vi "monitor.vi"(0 "HIFU_TCP in":refnum<k5>, 1 "HIFU":bool, 2 "chn num":i16=64, 3 "error in (no error)":errorcluster, 4 "sequence":u32) -> (5 "SEQ out":u32, 6 "current":dbl[](array[numeric]), 7 "HIFU_TCP out":refnum<k5>, 8 "voltage":dbl[](array[numeric]), 9 "OK?":bool, 10 "error out":errorcluster)   [LabVIEW 2016]
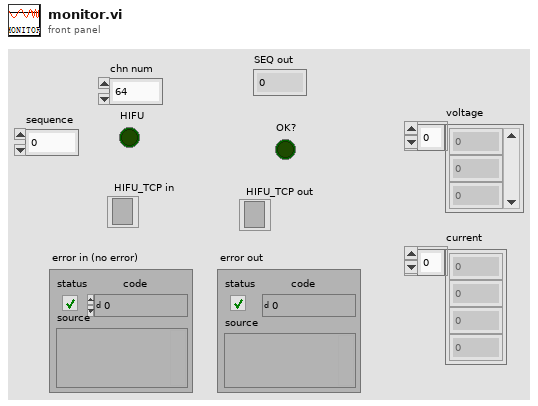
[diagram p1: front panel]
types:
  T1 = enum8{"SET_FREQ", "SET_VOLT", "SET_CHANNEL_VOLT", "SET_PHASE", "START_HEAT", "STOP_HEAT", "CHANNEL_CTRL_SINGLE", "CHANNEL_CTRL_ALL", "READ_VOLT_SET", "READ_VOLT_SET_RSP", "READ_CURRENT_VOLT", "READ_CURRENT_VOLT_RSP", "READ_PHASE", "READ_PHASE_RSP", "READ_HEATTIME_LEFT", "READ_HEATTIME_LEFT_RSP", "EXEC_RSP"}
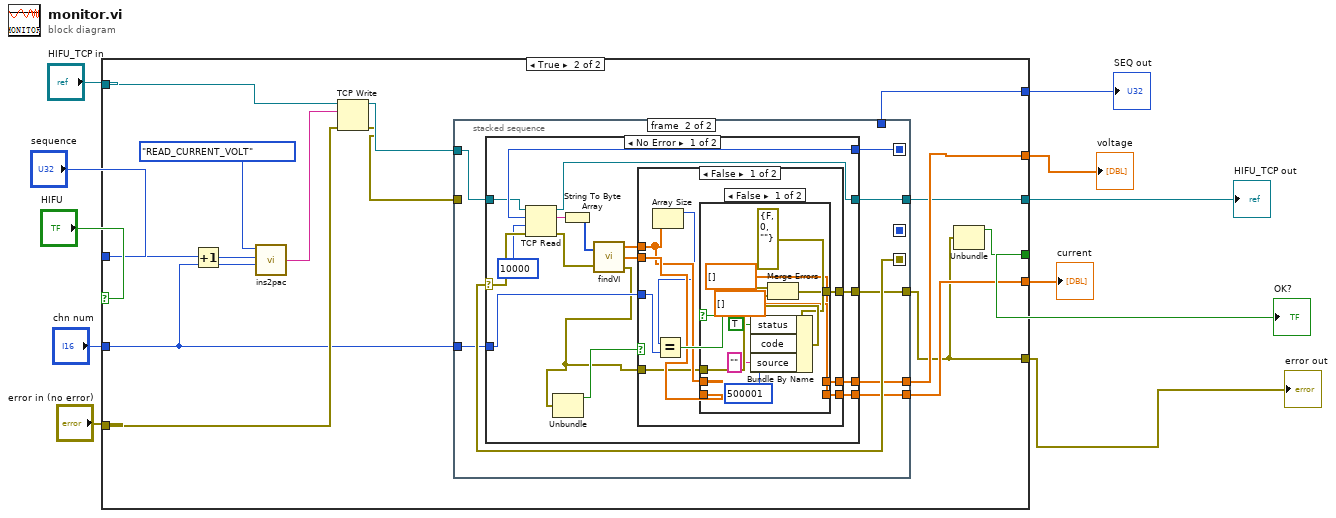
[diagram p0: block diagram]
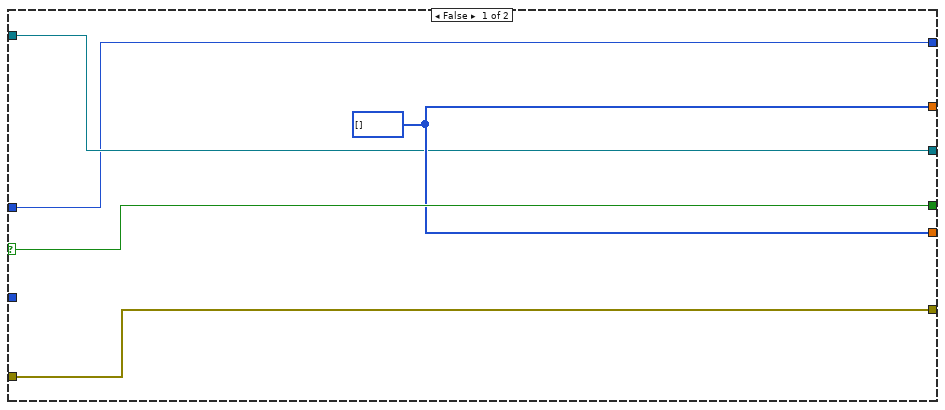
[diagram p2: hidden frame]
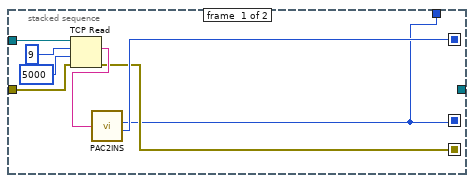
[diagram p3: hidden frame]
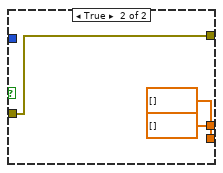
[diagram p5: hidden frame]
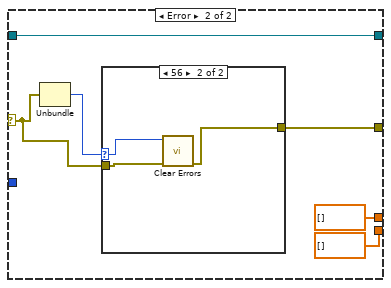
[diagram p6: hidden frame]
diagram:
  n1 = case shown="True" "HIFU" {
    selector: "HIFU" -> [w16 _]
    tunnel: "error in (no error)" -> [w15 w29]
    tunnel: [w14 w24] -> w9
    tunnel: [w14 w25] -> w8
    tunnel: [w15 w22] -> w1
    tunnel: [w16 w21] -> w7
    tunnel: "chn num" -> [_ w26]
    tunnel: "HIFU_TCP in" -> [w13 w31]
    tunnel: "sequence" -> [w12 w20]
    tunnel: [w13 w23] -> w3
    tunnel: [w12 w18] -> w2
    frame False {
      w14 = i32[] []
    }
    frame True {
      n2 = Increment(x=w20) -> (x+1=w19:u32)
      n3 = call "ins2pac.vi"("chn num"=w26, "SEQUENCE"=w19, "TYPE"=T1."READ_CURRENT_VOLT") -> ("PACKET"=w30:string)  [unwired: 1 in]
      n4 = TCP Write(connection ID=w31, data in=w30, error in (no error)=w29) -> (connection ID out=w28:refnum<k5>, error out=w27:errorcluster)  [unwired: 1 in, 1 out]
      n5 = stacked-sequence {
        seq-local: [w34 _] -> [_ w40]
        seq-local: [w32 _] -> [_ _]
        seq-local: [w33 _] -> [_ w46]
        tunnel: w28 -> [w39 w47]
        tunnel: w27 -> [w36 _]
        tunnel: w26 -> [_ w45]
        tunnel: [_ w44] -> w25
        tunnel: [_ w43] -> w24
        tunnel: [_ w42] -> w22
        tunnel: [_ w41] -> w23
        tunnel: [w32 _] -> w18
        frame #0 {
          n6 = TCP Read(connection ID=w39, bytes to read=9, error in (no error)=w36, 9:5000 ("timeout ms (25000)")) -> (data out=w35:string, error out=w33:errorcluster)  [unwired: 1 in, 1 out]
          n7 = call "PAC2INS.vi"("PACKET"=w35) -> ("SEQUENCE"=w32:u32, "LENGTH"=w34:u32)  [unwired: 2 out]
        }
        frame #1 {
          n8 = case shown="No Error" w46 {
            selector: w46 -> [w61 w89]
            tunnel: w40 -> [w63 _]
            tunnel: w47 -> [w62 w90]
            tunnel: w45 -> [w54 _]
            tunnel: [w53 dbl[] [] ("V")] -> w44
            tunnel: [w52 dbl[] [] ("I")] -> w43
            tunnel: [w51 w91] -> w42
            tunnel: [w50 w90] -> w41
            frame No Error {
              n9 = TCP Read(connection ID=w62, bytes to read=w63, error in (no error)=w61, 9:10000 ("timeout ms (25000)")) -> (connection ID out=w50:refnum<k5>, data out=w59:string, error out=w57:errorcluster)  [unwired: 1 in]
              n10 = String To Byte Array(string=w59) -> (unsigned byte array=w58:u8[])
              n11 = call "findVI.vi"("Array"=w58, "error in (no error)"=w57) -> ("V"=w56:dbl[], "I"=w55:dbl[], "error out"=w48:errorcluster)
              n12 = Unbundle(w48) -> ("status"=w49:bool)  [unwired: 2 out]
              n13 = case shown="False" w49 {
                tunnel: w56 -> [w69 _]
                tunnel: w55 -> [w70 _]
                tunnel: w54 -> [w72 _]
                tunnel: [w68 dbl[] [] ("V")] -> w53
                tunnel: [w67 dbl[] [] ("I")] -> w52
                tunnel: w48 -> [w66 w87]
                tunnel: [w65 w87] -> w51
                frame False {
                  n14 = Array Size(array=w69) -> (size(s)=w64:i32)
                  n15 = Equal?(x=w64, y=w72) -> (x = y?=w71:bool)
                  n16 = case shown="False" w71 {
                    tunnel: w70 -> [_ w83]
                    tunnel: w69 -> [_ w84]
                    tunnel: [dbl[] [] ("V") w84] -> w68
                    tunnel: [dbl[] [] ("I") w83] -> w67
                    tunnel: w66 -> [w81 w82]
                    tunnel: [w74 w82] -> w65
                    frame False {
                      n17 = Bundle By Name(cluster=errorcluster {"status"=FALSE, "code"=0, "source"=""} ("error constant"), "status"=TRUE, "code"=500001, "source"="") -> (w80:errorcluster)
                      n18 = Merge Errors(w81, w80) -> (w74:errorcluster)
                    }
                    frame True {
                    }
                  }
                }
                frame True {
                }
              }
            }
            frame Error {
              n19 = Unbundle(w89) -> ("code"=w88:i32)  [unwired: 2 out]
              n20 = case shown="56" w88 {
                selector: w88 -> [_ w97]
                tunnel: w89 -> [w94 w96]
                tunnel: [w94 w95] -> w91
                frame 0, Default {
                }
                frame 56 {
                  n21 = call <vilib>:"Clear Errors.vi"("error in (no error)"=w96, "specific error code to clear (0: all)"=w97) -> ("error out"=w95:errorcluster)  [unwired: 4 in, 1 out]
                }
              }
            }
          }
        }
      }
      n22 = Unbundle(w22) -> ("status"=w21:bool)  [unwired: 2 out]
    }
  }
  "error out" <- w1
  "voltage" <- w8
  "current" <- w9
  "OK?" <- w7
  "HIFU_TCP out" <- w3
  "SEQ out" <- w2
